vi "PC Take Data.vi"(8 "error in (no error)":errorcluster, 11 "Photon Counter SR400 in":refnum<class "Photon Counter SR400.lvclass">) -> (0 "error out":errorcluster, 1 "CPS B":dbl[unit], 2 "CPS A":dbl[unit], 3 "Photon Counter SR400 out":refnum<class "Photon Counter SR400.lvclass">)   [LabVIEW 2015, in "Photon Counter SR400.lvclass"]
uses:
  Photon Counter SR400.lvclass
  Photon Counter SR400.lvclass/Photon Counter SR400.ctl
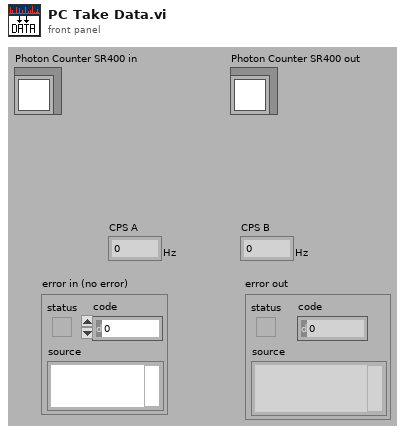
[diagram p1: front panel]
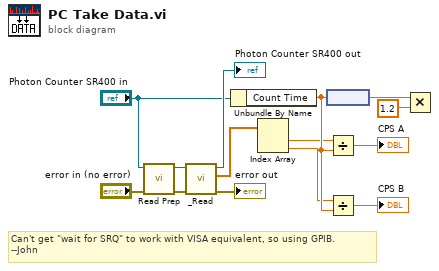
[diagram p0: block diagram]
diagram:
  # "Can't get \"wait for SRQ\" to work with VISA equivalent, so using GPIB. \n--John"
  n1 = call-dynamic "Read Prep.vi"("error in (no error)"="error in (no error)", "Photon Counter SR400 in"="Photon Counter SR400 in") -> ("error out"=w7:errorcluster, "Photon Counter SR400 out"=w9:refnum<class "Photon Counter SR400.lvclass">)  [unwired: 8 out]
  n2 = call-dynamic "_Read.vi"("error in (no error)"=w7, "Photon Counter SR400 in"=w9) -> ("error out"=→"error out":errorcluster, "4 Data Points"=w3:dbl[], "Photon Counter SR400 out"=→"Photon Counter SR400 out":refnum<class "Photon Counter SR400.lvclass">)  [unwired: 7 out]
  n3 = Unbundle By Name("Photon Counter SR400 in") -> ("Count Time"=w14:dbl[unit])
  n4 = Index Array(array=w3) -> (element #1=w2:dbl, element #2=w1:dbl)  [unwired: 2 in]
  n5 = node(w14) -> (w12:dbl)
  n6 = Divide(x=w2, y=w14) -> (x/y=→"CPS A":dbl[unit])
  n7 = Divide(x=w1, y=w14) -> (x/y=→"CPS B":dbl[unit])
  n8 = Multiply(x=w12, y=1.2) -> ()  [unwired: 1 out]
